vi "Continuous Serial Write and Read and plot.vi"(6 "Stop":bool, 8 "Command":string="*IDN?", 9 "XON/XOFF Characters":T1={"XON"=enum."DC1", "XOFF"=enum."DC3"}, 10 "Serial Settings":T3={"baud rate"=9600, "data bits"=8, "parity"=enum."None", "stop bits"=10, "flow control"=0} {"flow control" items=["None"=0, "XON/XOFF"=1, "RTS/CTS"=2, "DTR/DSR"=4]; "stop bits" items=["1.0"=10, "1.5"=15, "2.0"=20]; "data bits" min=5 max=8 step=1; "baud rate" items=["75"=75, "110"=110, "134"=134, "150"=150, "300"=300, "600"=600, "1200"=1200, "1800"=1800, "2400"=2400, "4800"=4800, "7200"=7200, "9600"=9600, "14400"=14400, "19200"=19200, "28800"=28800, "38400"=38400, "56000"=56000, "57600"=57600, "115200"=115200, "128000"=128000, "230400"=230400]}, 11 "VISA resource name":refnum<visa-resource-name>="COM1") -> (0 "Response":string, 3 "Waveform Chart":i32(graph))   [LabVIEW 2013]
doc: "This example performs writes and reads on a serial port, as directed by the user. You can press the Write and Read buttons, and change the Read Count, while the example is running.\n\nThe parameters set for the serial port must match the parameters of the connected instrument or device. In this example, the Read Count parameter specifies the number of bytes that the serial port reads. If there were more bytes at the port than the specified number, those bytes would not be read. If there were less bytes at the port than the specified number, you would receive a timeout error.\n\nThis example expands upon the flow control options for XON and XOFF, allowing the user to choose those control characters. Also, the user can enable or disable a termination character. Some devices require a termination character in order to identify the end of command strings. Some devices send a termination character to signify the end of data to be read. This example shows how you can end the Read operation once a termination character is detected in the buffer and/or append a termination character at the end of the Write data."
uses:
  Program Files/National Instruments/LabVIEW 2013/examples/Instrument IO/Serial/support/Serial - Settings.ctl
  Program Files/National Instruments/LabVIEW 2013/examples/Instrument IO/Serial/support/Serial - XON-XOFF Characters.ctl
  Program Files/National Instruments/LabVIEW 2013/examples/Instrument IO/Serial/support/Serial - ASCII Characters.ctl
  <vilib>/Instr/_visa.llb/VISA Configure Serial Port (Instr).vi
panel:
  in  "Read-Write":bool
  in  "Termination Character":u8=10 format="%.0x"
  in  "End Write on Termination Character?":bool=TRUE
  in  "Read Count":u32=1000
  in  "End Read on Termination Character?":bool=TRUE
  # "Overview: Demonstrates the use of the VISA functions to write commands to and read responses from a serial instrument continuously in a loop.\nRequirements: NI-VISA Driver\nInstructions:\n1. Run the VI.\n2. Specify a Command and click the Write button.\n3. Read a Response by clicking the Read button.\n4. Click Stop to stop the VI."
  # "0xA is equivalent to a '\\n' character, which is a line feed."
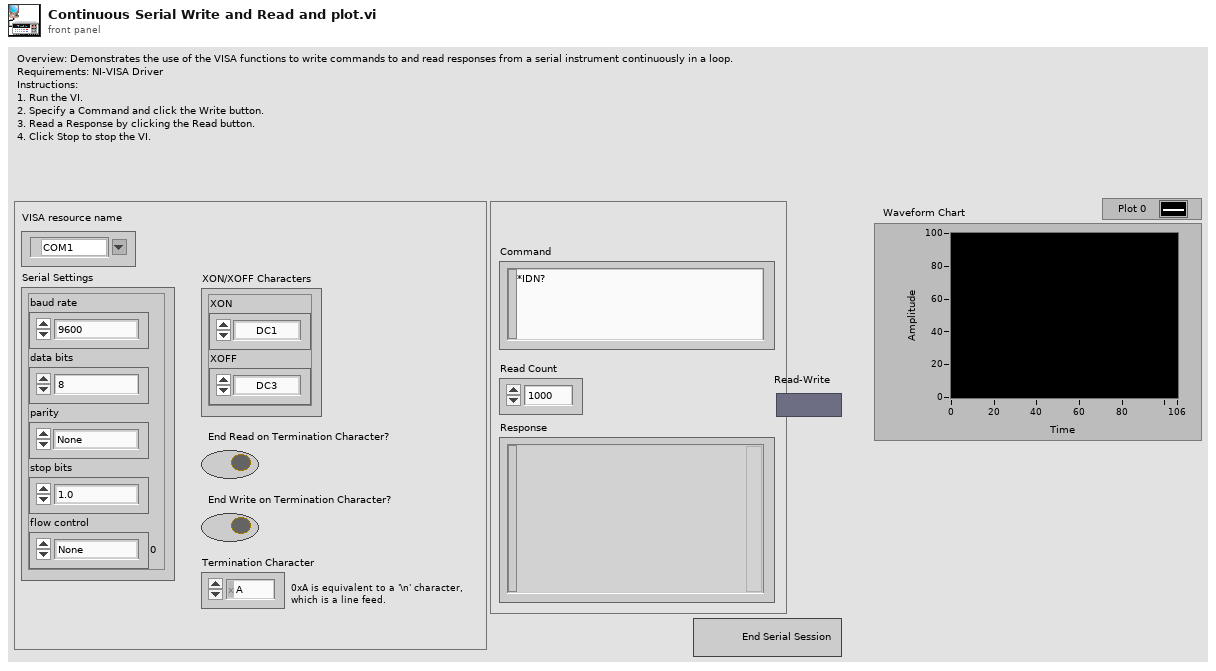
[diagram p1: front panel]
types:
  T1 = typedef "Serial - XON-XOFF Characters.ctl" = cluster{"XON":T2, "XOFF":T2}
  T2 = typedef "Serial - ASCII Characters.ctl" = enum16{"NUL", "SOH", "STX", "ETX", "EOT", "ENQ", "ACK", "BEL", "BS", "HT", "LF", "VT", "FF", "CR", "SO", "SI", "DLE", "DC1", "DC2", "DC3", "DC4", "NAK", "SYN", "ETB", "CAN", "EM", "SUB", "ESC", "FS", "GS", "RS", "US", "SP", "!", "\"", "#", "$", "%", "&", "'", "(", ")", "*", "+", ",", "- (-)", ".", "/", "0", "1", "2", "3", "4", "5", "6", "7", "8", "9", ":", ";", "<", "=", ">", "?", "@", "A", "B", "C", "D", "E", "F", "G", "H", "I", "J", "K", "L", "M", "N", "O", "P", "Q", "R", "S", "T", "U", "V", "W", "X", "Y", "Z", "[", "\\", "]", "^", "_", "`", "a", "b", "c", "d", "e", "f", "g", "h", "i", "j", "k", "l", "m", "n", "o", "p", "q", "r", "s", "t", "u", "v", "w", "x", "y", "z", "{", "|", "}", "~"}
  T3 = typedef "Serial - Settings.ctl" = cluster{"baud rate":u32, "data bits":u16, "parity":enum16{"None", "Odd", "Even", "Mark", "Space"}, "stop bits":u16, "flow control":u16}
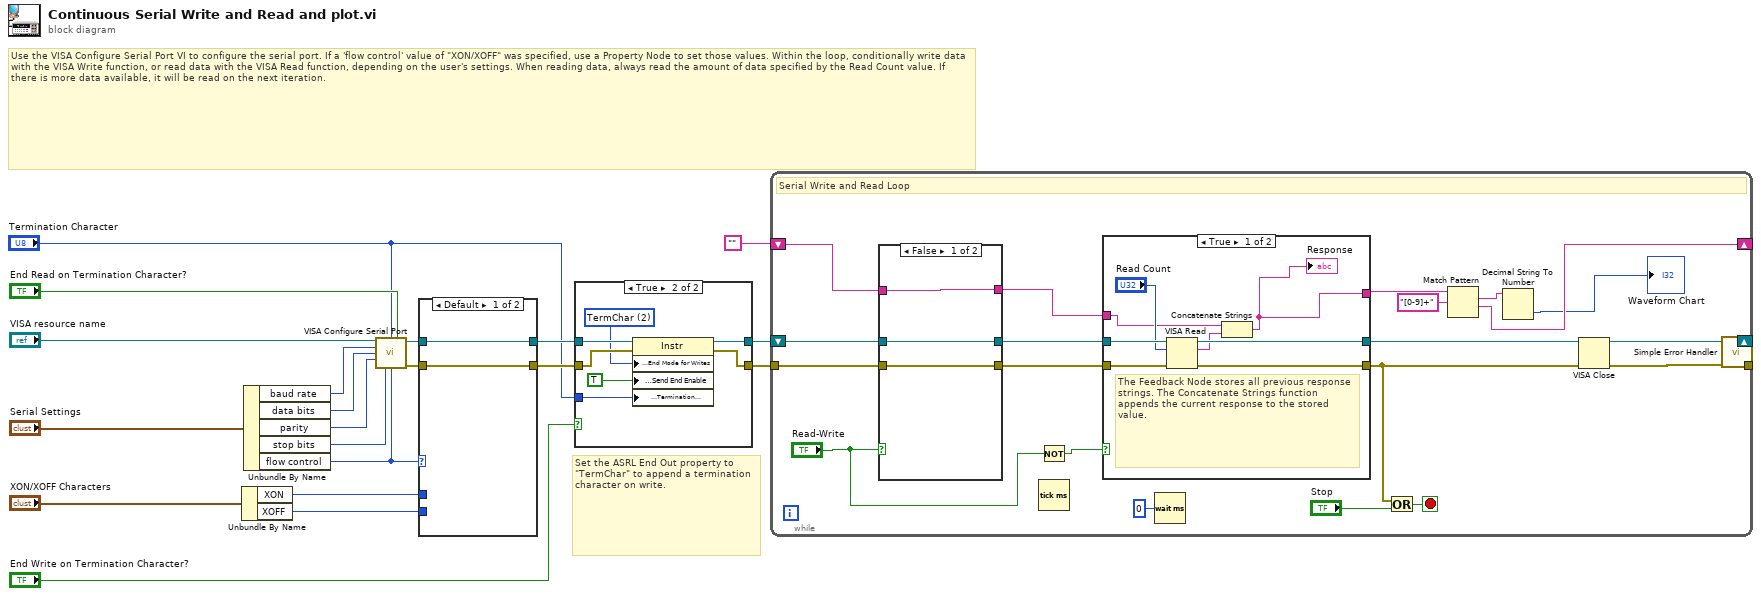
[diagram p0: block diagram]
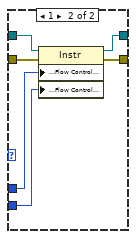
[diagram p3: hidden frame]
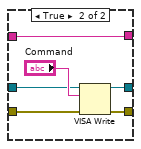
[diagram p4: hidden frame]
diagram:
  # "Set the ASRL End Out property to \"TermChar\" to append a termination character on write."
  # "Use the VISA Configure Serial Port VI to configure the serial port. If a 'flow control' value of \"XON/XOFF\" was specified, use a Property Node to set those values. Within the loop, conditionally write data with the VISA Write function, or read data with the VISA Read function, depending on the user's settings. When reading data, always read the amount of data specified by the Read Count value. If there is more data available, it will be read on the next iteration."
  n1 = Unbundle By Name("XON/XOFF Characters") -> ("XON"=w9:T2, "XOFF"=w8:T2)
  n2 = Unbundle By Name("Serial Settings") -> ("baud rate"=w16:u32, "data bits"=w17:u16, "parity"=w18:enum16{"None", "Odd", "Even", "Mark", "Space"}, "stop bits"=w19:u16, "flow control"=w10:u16)
  n3 = call-poly "VISA Configure Serial Port"("VISA resource name"="VISA resource name", "termination char\n(0xA = '\\n' = LF)"="Termination Character", "Enable Termination\nChar (T)"="End Read on Termination Character?", "baud rate (9600)"=w16, "data bits (8)"=w17, "parity (0:none)"=w18, "stop bits (10: 1 bit)"=w19, "flow control (0:none)"=w10) -> ("VISA resource name out"=w20:refnum<visa-resource-name>, "error out"=w21:errorcluster)  [unwired: 2 in, 4 out]
  n4 = case shown="Default" w10 {
    tunnel: [w24 w31] -> w7
    tunnel: [w25 w30] -> w5
    tunnel: w21 -> [w24 w29]
    tunnel: w20 -> [w25 w28]
    tunnel: w9 -> [_ w27]
    tunnel: w8 -> [_ w26]
    frame Default {
    }
    frame 1 {
      n5 = property class="Instr"(reference=w28, error in=w29, "Serial Settings:Flow Control XON Character"=w27, "Serial Settings:Flow Control XOFF Character"=w26) -> (reference out=w30:refnum<visa-resource-name>, error out=w31:errorcluster)
    }
  }
  n6 = case shown="True" "End Write on Termination Character?" {
    tunnel: w5 -> [w32 w40]
    tunnel: w7 -> [w33 w39]
    tunnel: [w32 w38] -> w4
    tunnel: [w33 w37] -> w6
    tunnel: "Termination Character" -> [_ w35]
    frame False {
    }
    frame True {
      w36 = u16 2 items=["None", "LastBit", "TermChar", "Break"] ("Serial Settings:Serial End Mode for Writes")
      n7 = property class="Instr"(reference=w40, error in=w39, "Serial Settings:End Mode for Writes"=w36, "Message Based Settings:Send End Enable"=TRUE, "Message Based Settings:Termination Character"=w35) -> (reference out=w38:refnum<visa-resource-name>, error out=w37:errorcluster)
    }
  }
  n8 = while {
    shift-right: [w58] -> w11
    shift-left: w4 -> [w57]
    tunnel: w6 -> [w56]
    tunnel: [w51] -> w12
    shift-right: [w44] -> _
    shift-left: "" -> [w46]
    stop <- w52 stop-if-true
    # "Serial Write and Read Loop"
    n9 = case shown="False" "Read-Write" {
      tunnel: w57 -> [w61 w66]
      tunnel: w56 -> [w60 w65]
      tunnel: [w61 w64] -> w55
      tunnel: [w60 w63] -> w54
      tunnel: w46 -> [w59 w62]
      tunnel: [w59 w62] -> w45
      frame False {
      }
      frame True {
        n10 = VISA Write(VISA resource name=w66, write buffer="Command", error in (no error)=w65) -> (VISA resource name out=w64:refnum<visa-resource-name>, error out=w63:errorcluster)  [unwired: 1 out]
      }
    }
    n11 = Not(x="Read-Write") -> (.not. x?=w43:bool)
    n12 = Tick Count (ms)() -> ()  [unwired: 1 out]
    n13 = case shown="True" w43 {
      tunnel: [w73 w78] -> w58
      tunnel: w55 -> [w75 w78]
      tunnel: [w71 w77] -> w51
      tunnel: w54 -> [w74 w77]
      tunnel: [w68 w76] -> w49
      tunnel: w45 -> [w69 w76]
      frame True {
        # "The Feedback Node stores all previous response strings. The Concatenate Strings function appends the current response to the stored value."
        n14 = VISA Read(VISA resource name=w75, byte count="Read Count", error in (no error)=w74) -> (VISA resource name out=w73:refnum<visa-resource-name>, read buffer=w70:string, error out=w71:errorcluster)  [unwired: 1 out]
        n15 = Concatenate Strings(w69, w70) -> (w68:string)
        "Response" <- w68
      }
      frame False {
      }
    }
    n16 = Wait (ms)(milliseconds to wait=u32 0) -> ()  [unwired: 1 out]
    n17 = Or(x=w51, y="Stop") -> (x .or. y?=w52:bool)
    n18 = Match Pattern(string=w49, regular expression="[0-9]+") -> (match substring=w47:string, after substring=w44:string)  [unwired: 1 in, 2 out]
    n19 = Decimal String To Number(string=w47) -> (number=→"Waveform Chart":i32)  [unwired: 2 in, 1 out]
  }
  n20 = VISA Close(VISA resource name=w11, error in (no error)=w12) -> (error out=w13:errorcluster)
  n21 = call <vilib>:"Simple Error Handler.vi"("error in (no error)"=w13) -> ()  [unwired: 1 in, 8 out]
